vi "from string.vi"(8 "error in":errorcluster, 9 "data":string, 10 "version":string, 11 "Shared Memory configuration in":refnum<class "Shared Memory configuration.lvclass">) -> (0 "error out":errorcluster, 3 "Shared Memory configuration out":refnum<class "Shared Memory configuration.lvclass">)   [LabVIEW 2014, in "Shared Memory configuration.lvclass"]
doc: "Provides an interface for loading a module configuration from a file or other serialized data source. It is recommended that all children of this class store data in two sets--data required for its own initialization, and any data required for parent initialization--and that each implementation uses the <b>Call Parent Method</b> primitive to de-serialize parent information. As a result, it is expected that every module configuration class calls <b>component configuration.lvclass:From String.vi</b>."
uses:
  Shared Memory configuration.lvclass
  <vilib>/NI/Tag Bus Module Framework/module configuration/TBM module configuration.lvclass
  <vilib>/NI/Configuration Framework/serializable configuration/NISE_CEF_serializable configuration.lvclass
  <vilib>/NI/Tag Bus Module Framework/channel/TBM channel.lvclass
  Line.ctl
  editor node/sync/sync mechanism.ctl
  editor node/sync/sync item.ctl
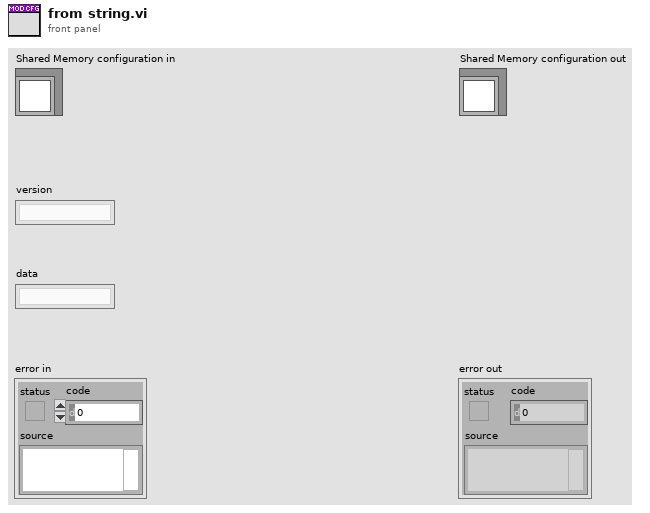
[diagram p1: front panel]
types:
  T1 = typedef "Shared Memory configuration.lvclass/Line.ctl" = cluster{"channel":refnum<class "TBM channel.lvclass">}
  T2 = typedef "Shared Memory configuration.lvclass/sync item.ctl" = cluster{"mechanism":T3, "name":string}
  T3 = typedef "Shared Memory configuration.lvclass/sync mechanism.ctl" = enum16{"Semaphore"}
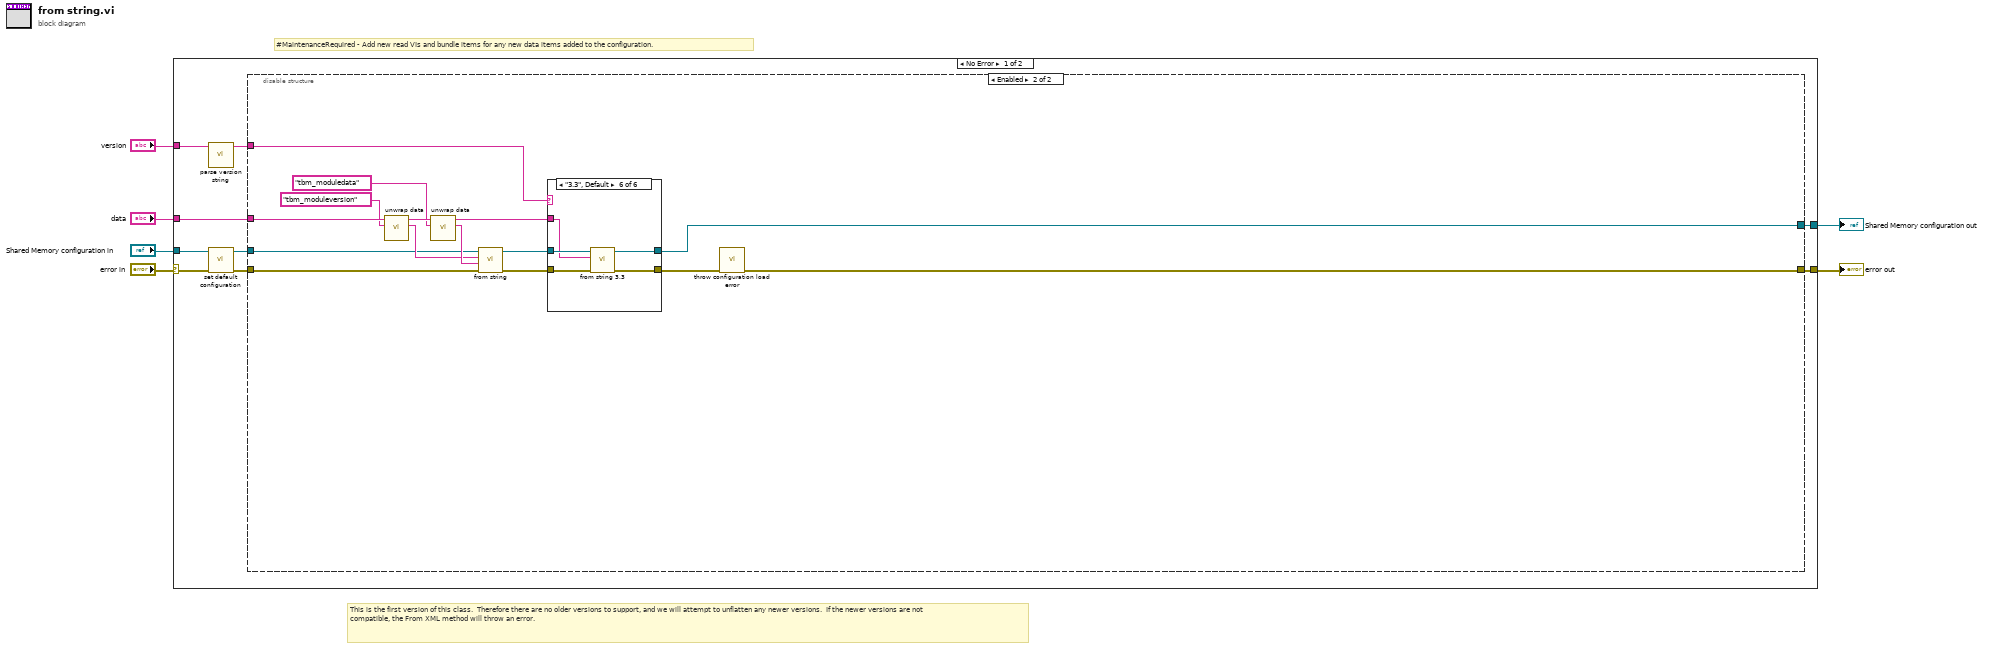
[diagram p0: block diagram]
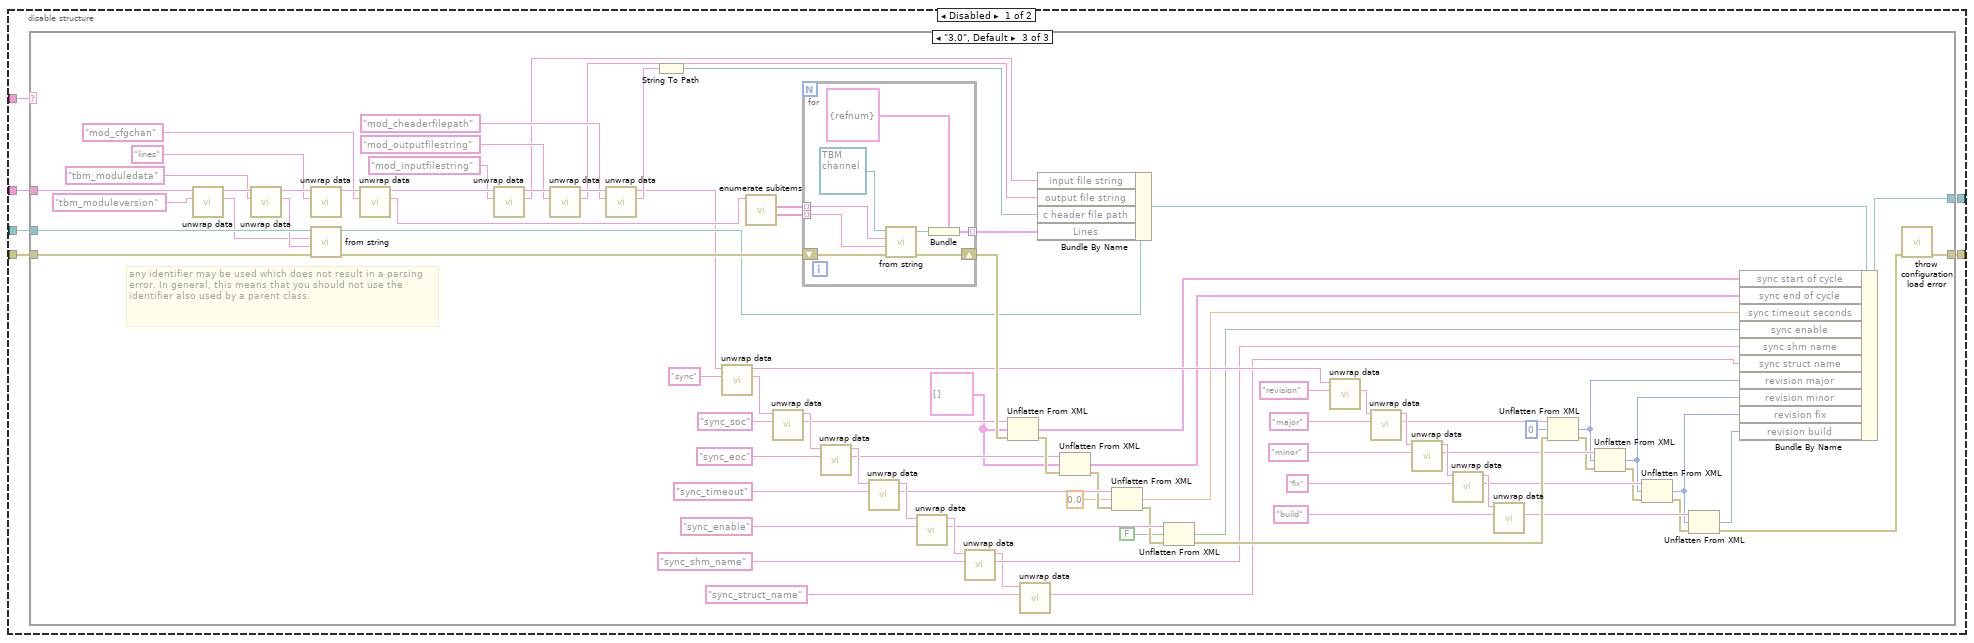
[diagram p2: hidden frame]
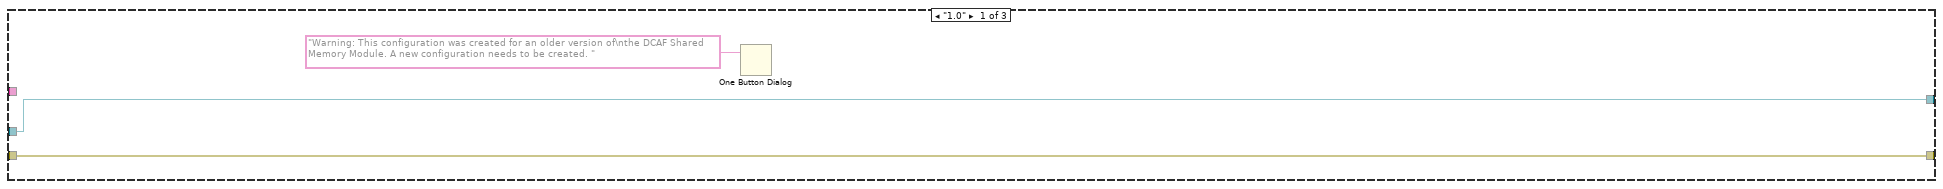
[diagram p3: hidden frame]
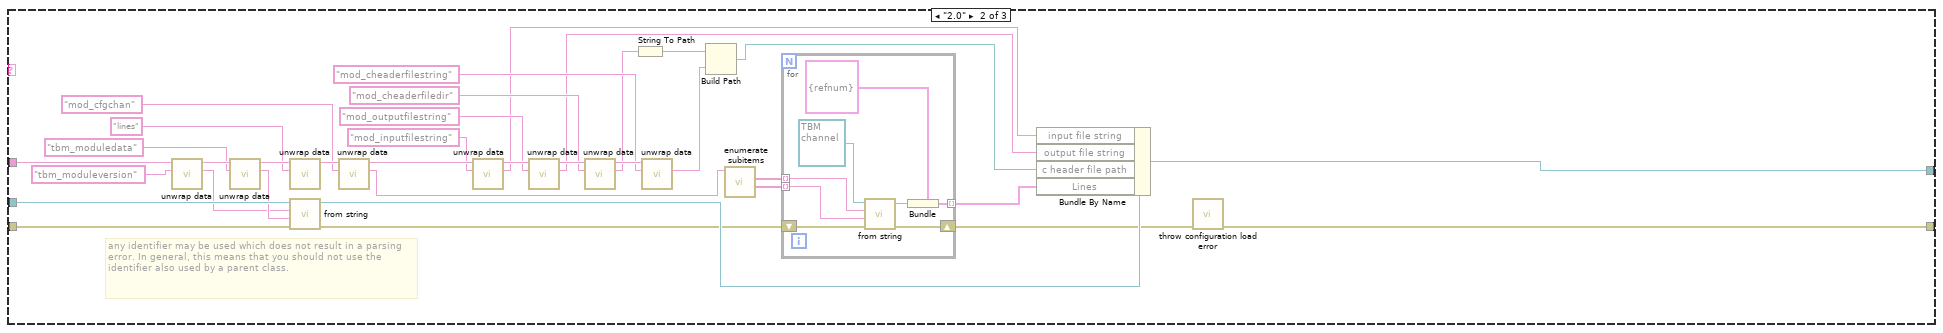
[diagram p4: hidden frame]
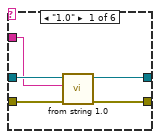
[diagram p5: hidden frame]
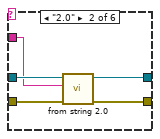
[diagram p6: hidden frame]
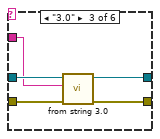
[diagram p7: hidden frame]
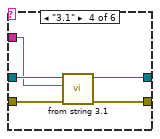
[diagram p8: hidden frame]
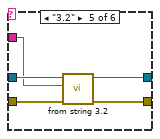
[diagram p9: hidden frame]
diagram:
  # "#MaintenanceRequired - Add new read VIs and bundle items for any new data items added to the configuration."
  # "This is the first version of this class.  Therefore there are no older versions to support, and we will attempt to unflatten any newer versions.  If the newer versions are not compatible, the From XML method will throw an error."
  n1 = case shown="No Error" "error in" {
    selector: "error in" -> [w9 w208]
    tunnel: "data" -> [w15 _]
    tunnel: "Shared Memory configuration in" -> [w10 w207]
    tunnel: [w14 w207] -> w5
    tunnel: [w13 w208] -> w4
    tunnel: "version" -> [w12 _]
    frame No Error {
      n2 = call <vilib>:"parse version string.vi"("full version"=w12) -> ("major.minor version"=w11:string)  [unwired: 7 in, 3 out]
      n3 = call "set default configuration.vi"("error in"=w9, "Shared Memory configuration in"=w10) -> ("error out"=w8:errorcluster, "Shared Memory configuration out"=w7:refnum<class "Shared Memory configuration.lvclass">)  [unwired: 8 in]
      n4 = disable-structure shown="Enabled" {
        disable-tunnel: w15 -> [w21 w173]
        disable-tunnel: [w20 w162] -> w14
        disable-tunnel: [w19 w163] -> w13
        disable-tunnel: w11 -> [w18 w164]
        disable-tunnel: w8 -> [w17 w170]
        disable-tunnel: w7 -> [w16 w169]
        frame Disabled {
          n5 = case shown="\"3.0\", Default" w18 {
            tunnel: w21 -> [_ w56 w147]
            tunnel: w17 -> [w24 w55 w146]
            tunnel: w16 -> [w23 w59 w150]
            tunnel: [w23 w47 w109] -> w20
            tunnel: [w24 w58 w149] -> w19
            frame "1.0" {
              n6 = One Button Dialog(message="Warning: This configuration was created for an older version of\nthe DCAF Shared Memory Module. A new configuration needs to be created. ") -> ()  [unwired: 1 in, 1 out]
            }
            frame "2.0" {
              # "any identifier may be used which does not result in a parsing error. In general, this means that you should not use the identifier also used by a parent class."
              n7 = call <vilib>:"unwrap data.vi"("identifier"="tbm_moduleversion" ("additional identifier"), "data to unwrap"=w56) -> ("unwrapped data"=w51:string, "remaining string"=w57:string)  [unwired: 8 in]
              n8 = call <vilib>:"unwrap data.vi"("identifier"="tbm_moduledata" ("additional identifier"), "data to unwrap"=w57) -> ("unwrapped data"=w53:string, "remaining string"=w50:string)  [unwired: 8 in]
              n9 = call <vilib>:"unwrap data.vi"("identifier"="lines" ("additional identifier"), "data to unwrap"=w50) -> ("remaining string"=w46:string)  [unwired: 8 in, 1 out]
              n10 = call-parent "from string.vi"("error in"=w55, "data"=w53, "version"=w51, "module configuration in"=w59) -> ("error out"=w42:errorcluster, "module configuration out"=w48:refnum<class "Shared Memory configuration.lvclass">)  [unwired: 6 in]
              n11 = call <vilib>:"unwrap data.vi"("identifier"="mod_cfgchan", "data to unwrap"=w46) -> ("unwrapped data"=w41:string, "remaining string"=w38:string)  [unwired: 8 in]
              n12 = call <vilib>:"unwrap data.vi"("identifier"="mod_inputfilestring", "data to unwrap"=w38) -> ("unwrapped data"=w30:string, "remaining string"=w37:string)  [unwired: 8 in]
              n13 = call <vilib>:"unwrap data.vi"("identifier"="mod_outputfilestring", "data to unwrap"=w37) -> ("unwrapped data"=w29:string, "remaining string"=w36:string)  [unwired: 8 in]
              n14 = call <vilib>:"unwrap data.vi"("identifier"="mod_cheaderfiledir", "data to unwrap"=w36) -> ("unwrapped data"=w28:string, "remaining string"=w35:string)  [unwired: 8 in]
              n15 = String To Path(string=w28) -> (path=w26:path)
              n16 = call <vilib>:"unwrap data.vi"("identifier"="mod_cheaderfilestring", "data to unwrap"=w35) -> ("unwrapped data"=w27:string)  [unwired: 8 in, 1 out]
              n17 = Build Path(base path=w26, name or relative path=w27) -> (appended path=w25:path)
              n18 = call <vilib>:"enumerate subitems.vi"("data to enumerate"=w41) -> ("associated data"=w43:string[], "discovered subitems"=w44:string[])  [unwired: 8 in, 1 out]
              n19 = for {
                shift-right: [w67] -> w39
                shift-left: w42 -> [w66]
                tunnel: w44 -> [w65] mode=indexing
                tunnel: w43 -> [w64] mode=indexing
                tunnel: [w60] -> w40 mode=indexing
                n20 = call-dynamic "from string.vi"("error in"=w66, "channel data"=w64, "identifier"=w65, "channel in"=refnum<class "TBM channel.lvclass"> refnum) -> ("error out"=w67:errorcluster, "channel out"=w61:refnum<class "TBM channel.lvclass">)  [unwired: 6 in]
                n21 = Bundle(cluster=T1 {"channel"=refnum} ("Line"), "channel"=w61) -> (w60:T1)
              }
              n22 = Bundle By Name(cluster=w48, "input file string"=w30, "output file string"=w29, "c header file path"=w25, "Lines"=w40) -> (w47:refnum<class "Shared Memory configuration.lvclass">)
              n23 = call <vilib>:"throw configuration load error.vi"("error in"=w39) -> ("error out"=w58:errorcluster)  [unwired: 10 in]
            }
            frame "3.0", Default {
              w106 = T2[] [] ("sync start of cycle")
              # "any identifier may be used which does not result in a parsing error. In general, this means that you should not use the identifier also used by a parent class."
              n24 = call <vilib>:"unwrap data.vi"("identifier"="tbm_moduleversion" ("additional identifier"), "data to unwrap"=w147) -> ("unwrapped data"=w142:string, "remaining string"=w148:string)  [unwired: 8 in]
              n25 = call <vilib>:"unwrap data.vi"("identifier"="tbm_moduledata" ("additional identifier"), "data to unwrap"=w148) -> ("unwrapped data"=w144:string, "remaining string"=w141:string)  [unwired: 8 in]
              n26 = call <vilib>:"unwrap data.vi"("identifier"="lines" ("additional identifier"), "data to unwrap"=w141) -> ("remaining string"=w139:string)  [unwired: 8 in, 1 out]
              n27 = call-parent "from string.vi"("error in"=w146, "data"=w144, "version"=w142, "module configuration in"=w150) -> ("error out"=w136:errorcluster, "module configuration out"=w111:refnum<class "Shared Memory configuration.lvclass">)  [unwired: 6 in]
              n28 = call <vilib>:"unwrap data.vi"("identifier"="mod_cfgchan", "data to unwrap"=w139) -> ("unwrapped data"=w135:string, "remaining string"=w133:string)  [unwired: 8 in]
              n29 = call <vilib>:"unwrap data.vi"("identifier"="mod_inputfilestring", "data to unwrap"=w133) -> ("unwrapped data"=w124:string, "remaining string"=w132:string)  [unwired: 8 in]
              n30 = call <vilib>:"unwrap data.vi"("identifier"="mod_outputfilestring", "data to unwrap"=w132) -> ("unwrapped data"=w127:string, "remaining string"=w131:string)  [unwired: 8 in]
              n31 = call <vilib>:"unwrap data.vi"("identifier"="mod_cheaderfilepath", "data to unwrap"=w131) -> ("unwrapped data"=w126:string, "remaining string"=w72:string)  [unwired: 8 in]
              n32 = String To Path(string=w126) -> (path=w125:path)
              n33 = call <vilib>:"unwrap data.vi"("identifier"="sync", "data to unwrap"=w72) -> ("unwrapped data"=w115:string, "remaining string"=w121:string)  [unwired: 8 in]
              n34 = call <vilib>:"enumerate subitems.vi"("data to enumerate"=w135) -> ("associated data"=w137:string[], "discovered subitems"=w138:string[])  [unwired: 8 in, 1 out]
              n35 = call <vilib>:"unwrap data.vi"("identifier"="sync_soc", "data to unwrap"=w115) -> ("unwrapped data"=w108:string, "remaining string"=w114:string)  [unwired: 8 in]
              n36 = for {
                shift-right: [w161] -> w152
                shift-left: w136 -> [w160]
                tunnel: w138 -> [w159] mode=indexing
                tunnel: w137 -> [w158] mode=indexing
                tunnel: [w154] -> w134 mode=indexing
                n37 = call-dynamic "from string.vi"("error in"=w160, "channel data"=w158, "identifier"=w159, "channel in"=refnum<class "TBM channel.lvclass"> refnum) -> ("error out"=w161:errorcluster, "channel out"=w155:refnum<class "TBM channel.lvclass">)  [unwired: 6 in]
                n38 = Bundle(cluster=T1 {"channel"=refnum} ("Line"), "channel"=w155) -> (w154:T1)
              }
              n39 = call <vilib>:"unwrap data.vi"("identifier"="sync_eoc", "data to unwrap"=w114) -> ("unwrapped data"=w107:string, "remaining string"=w113:string)  [unwired: 8 in]
              n40 = call <vilib>:"unwrap data.vi"("identifier"="sync_timeout", "data to unwrap"=w113) -> ("unwrapped data"=w105:string, "remaining string"=w112:string)  [unwired: 8 in]
              n41 = call <vilib>:"unwrap data.vi"("identifier"="sync_enable", "data to unwrap"=w112) -> ("unwrapped data"=w103:string, "remaining string"=w104:string)  [unwired: 8 in]
              n42 = call <vilib>:"unwrap data.vi"("identifier"="sync_shm_name", "data to unwrap"=w104) -> ("unwrapped data"=w94:string, "remaining string"=w70:string)  [unwired: 8 in]
              n43 = Unflatten From XML(xml string=w108, type=w106, error in (no error)=w152) -> (value=w98:T2[], error out=w151:errorcluster)
              n44 = call <vilib>:"unwrap data.vi"("identifier"="sync_struct_name", "data to unwrap"=w70) -> ("unwrapped data"=w69:string)  [unwired: 8 in, 1 out]
              n45 = Bundle By Name(cluster=w111, "input file string"=w124, "output file string"=w127, "c header file path"=w125, "Lines"=w134) -> (w110:refnum<class "Shared Memory configuration.lvclass">)
              n46 = Unflatten From XML(xml string=w107, type=w106, error in (no error)=w151) -> (value=w97:T2[], error out=w102:errorcluster)
              n47 = Unflatten From XML(xml string=w105, type=0.0, error in (no error)=w102) -> (value=w96:dbl, error out=w101:errorcluster)
              n48 = Unflatten From XML(xml string=w103, type=FALSE, error in (no error)=w101) -> (value=w95:bool, error out=w153:errorcluster)
              n49 = call <vilib>:"unwrap data.vi"("identifier"="revision", "data to unwrap"=w121) -> ("unwrapped data"=w73:string)  [unwired: 8 in, 1 out]
              n50 = call <vilib>:"unwrap data.vi"("identifier"="major", "data to unwrap"=w73) -> ("unwrapped data"=w87:string, "remaining string"=w93:string)  [unwired: 8 in]
              n51 = call <vilib>:"unwrap data.vi"("identifier"="minor", "data to unwrap"=w93) -> ("unwrapped data"=w88:string, "remaining string"=w92:string)  [unwired: 8 in]
              n52 = call <vilib>:"unwrap data.vi"("identifier"="fix", "data to unwrap"=w92) -> ("unwrapped data"=w89:string, "remaining string"=w91:string)  [unwired: 8 in]
              n53 = call <vilib>:"unwrap data.vi"("identifier"="build", "data to unwrap"=w91) -> ("unwrapped data"=w90:string)  [unwired: 8 in, 1 out]
              n54 = Unflatten From XML(xml string=w87, type=u8 0, error in (no error)=w153) -> (value=w77:u8, error out=w82:errorcluster)
              n55 = Unflatten From XML(xml string=w88, type=w77, error in (no error)=w82) -> (value=w76:u8, error out=w81:errorcluster)
              n56 = Unflatten From XML(xml string=w89, type=w76, error in (no error)=w81) -> (value=w75:u8, error out=w80:errorcluster)
              n57 = Unflatten From XML(xml string=w90, type=w75, error in (no error)=w80) -> (value=w74:u8, error out=w78:errorcluster)
              n58 = Bundle By Name(cluster=w110, "sync start of cycle"=w98, "sync end of cycle"=w97, "sync timeout seconds"=w96, "sync enable"=w95, "sync shm name"=w94, "sync struct name"=w69, "revision major"=w77, "revision minor"=w76, "revision fix"=w75, "revision build"=w74) -> (w109:refnum<class "Shared Memory configuration.lvclass">)
              n59 = call <vilib>:"throw configuration load error.vi"("error in"=w78) -> ("error out"=w149:errorcluster)  [unwired: 10 in]
            }
          }
        }
        frame Enabled {
          n60 = call <vilib>:"unwrap data.vi"("identifier"="tbm_moduleversion" ("additional identifier"), "data to unwrap"=w173) -> ("unwrapped data"=w171:string, "remaining string"=w176:string)  [unwired: 8 in]
          n61 = call <vilib>:"unwrap data.vi"("identifier"="tbm_moduledata" ("additional identifier"), "data to unwrap"=w176) -> ("unwrapped data"=w174:string, "remaining string"=w166:string)  [unwired: 8 in]
          n62 = call-parent "from string.vi"("error in"=w170, "data"=w174, "version"=w171, "module configuration in"=w169) -> ("error out"=w168:errorcluster, "module configuration out"=w167:refnum<class "Shared Memory configuration.lvclass">)  [unwired: 6 in]
          n63 = case shown="\"3.3\", Default" w164 {
            tunnel: w168 -> [w181 w186 w190 w196 w200 w206]
            tunnel: w167 -> [w180 w185 w189 w193 w198 w204]
            tunnel: w166 -> [w179 w184 w187 w192 w197 w202]
            tunnel: [w177 w183 w191 w195 w201 w205] -> w165
            tunnel: [w178 w182 w188 w194 w199 w203] -> w162
            frame "1.0" {
              n64 = call "from string 1.0.vi"("error in"=w181, "data in"=w179, "Shared Memory configuration in"=w180) -> ("error out"=w177:errorcluster, "Shared Memory configuration out"=w178:refnum<class "Shared Memory configuration.lvclass">)  [unwired: 6 in, 1 out]
            }
            frame "2.0" {
              n65 = call "from string 2.0.vi"("error in"=w186, "data in"=w184, "Shared Memory configuration in"=w185) -> ("error out"=w183:errorcluster, "Shared Memory configuration out"=w182:refnum<class "Shared Memory configuration.lvclass">)  [unwired: 6 in, 1 out]
            }
            frame "3.0" {
              n66 = call "from string 3.0.vi"("error in"=w190, "data in"=w187, "Shared Memory configuration in"=w189) -> ("error out"=w191:errorcluster, "Shared Memory configuration out"=w188:refnum<class "Shared Memory configuration.lvclass">)  [unwired: 6 in, 1 out]
            }
            frame "3.1" {
              n67 = call "from string 3.1.vi"("error in"=w196, "data in"=w192, "Shared Memory configuration in"=w193) -> ("error out"=w195:errorcluster, "Shared Memory configuration out"=w194:refnum<class "Shared Memory configuration.lvclass">)  [unwired: 6 in, 1 out]
            }
            frame "3.2" {
              n68 = call "from string 3.2.vi"("error in"=w200, "data in"=w197, "Shared Memory configuration in"=w198) -> ("error out"=w201:errorcluster, "Shared Memory configuration out"=w199:refnum<class "Shared Memory configuration.lvclass">)  [unwired: 6 in, 1 out]
            }
            frame "3.3", Default {
              n69 = call "from string 3.3.vi"("error in"=w206, "data in"=w202, "Shared Memory configuration in"=w204) -> ("error out"=w205:errorcluster, "Shared Memory configuration out"=w203:refnum<class "Shared Memory configuration.lvclass">)  [unwired: 6 in, 1 out]
            }
          }
          n70 = call <vilib>:"throw configuration load error.vi"("error in"=w165) -> ("error out"=w163:errorcluster)  [unwired: 10 in]
        }
      }
    }
    frame Error {
    }
  }
  "error out" <- w4
  "Shared Memory configuration out" <- w5
